vi "Test Set Active Funnel.vi"(8 "error in (no error)":errorcluster) -> (0 "error out":errorcluster)   [LabVIEW 2019]
uses:
  <vilib>/addons/_JKI Toolkits/Caraya/classes/Test/Test.lvclass
  <vilib>/addons/_JKI Toolkits/Caraya/classes/Assert/Assert.lvclass
  Setting Database/Setting Database.lvclass
  <vilib>/JKI/JKI SMO/SMO/SMO.lvclass
  C:/Program Files (x86)/National Instruments/LabVIEW 2019/vi.lib/JKI/JKI SMO/SMO/SMO.lvclass
  Funnel Settings/Funnel Settings.lvclass
  C:/Users/Albro/Documents/GitHub/AFM-Lithography/lvsrc/Classes/Settings/ObjectSettings/ObjectSettings.lvclass
  <vilib>/addons/_JKI Toolkits/Caraya/classes/Assert/Assert Equal Value_Variant.vi
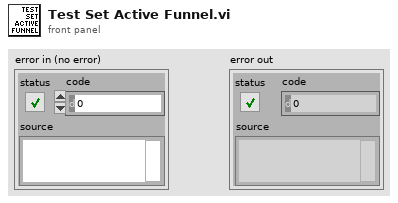
[diagram p1: front panel]
types:
  T1 = typedef "Setting Database.lvclass/PublicEvents--Cluster.ctl" = cluster{"NewActivePath":refnum<user-event>, "PathsUpdated":refnum<user-event>, "RectanglesUpdated":refnum<user-event>, "NewActiveRectangle":refnum<user-event>, "NewActiveFunnel":refnum<user-event>, "FunnelsUpdated":refnum<user-event>, "NewActiveDot":refnum<user-event>, "DotsUpdated":refnum<user-event>}
  T2 = typedef "Setting Database.lvclass/PrivateEvents--Setting Database.Refresh.ctl" = cluster{"Paths":string[], "Rectangles":string[], "Funnels":string[], "Dots":string[]}
  T3 = typedef "Setting Database.lvclass/PublicEvents--Setting Database.NewActiveFunnel.ctl" = refnum<class "Funnel Settings.lvclass">
  T4 = typedef "Setting Database.lvclass/PublicEvents--Setting Database.FunnelsUpdated.ctl" = refnum<class "Funnel Settings.lvclass">[]
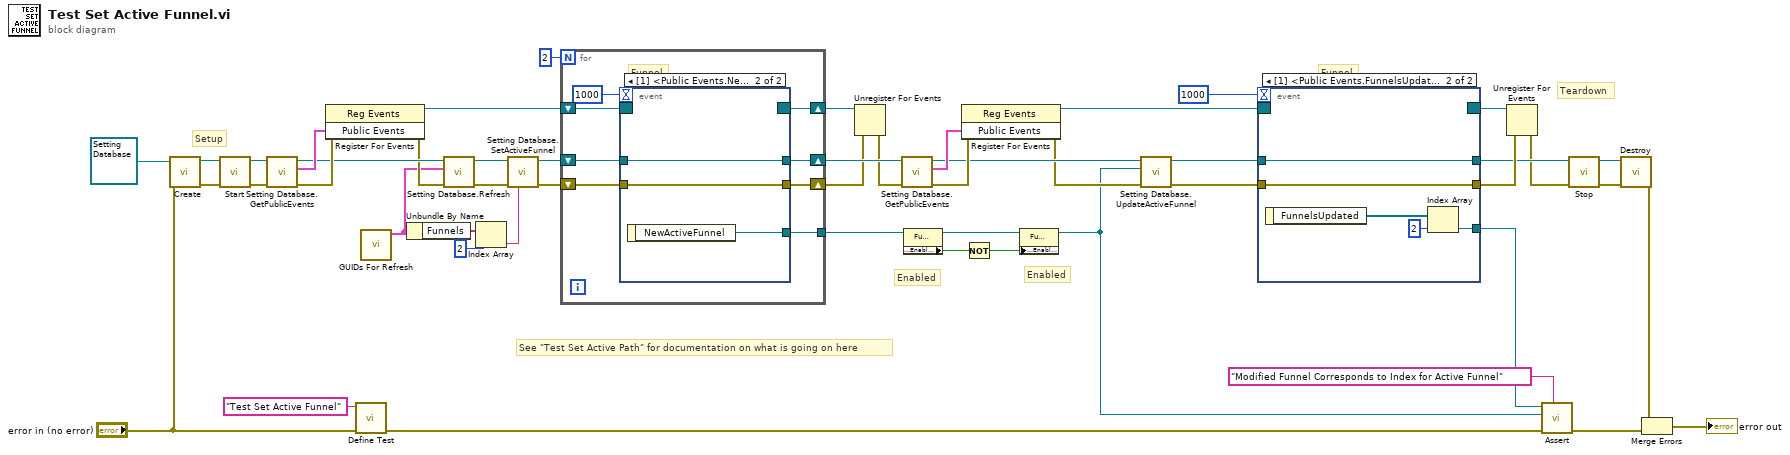
[diagram p0: block diagram]
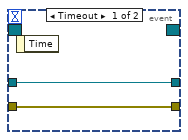
[diagram p2: hidden frame]
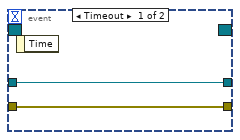
[diagram p3: hidden frame]
diagram:
  # "See \"Test Set Active Path\" for documentation on what is going on here"
  # "Enabled"
  # "Enabled"
  # "Funnel"
  # "Teardown"
  # "Setup"
  n1 = call <vilib>:"Create.vi"("error in (no error)"="error in (no error)", "SMO"=refnum<class "Setting Database.lvclass"> refnum ("Setting Database.lvclass")) -> ("error out"=w47:errorcluster, "SMO out"=w40:refnum<class "Setting Database.lvclass">)  [unwired: 7 in, 1 out]
  n2 = call <vilib>:"Start.vi"("error in (no error)"=w47, "SMO"=w40) -> ("error out"=w46:errorcluster, "SMO out"=w39:refnum<class "Setting Database.lvclass">)  [unwired: 8 in]
  n3 = call "Setting Database.GetPublicEvents.vi"("error in (no error)"=w46, "Setting Database"=w39) -> ("error out"=w44:errorcluster, "Public Events"=w36:T1, "Setting Database out"=w33:refnum<class "Setting Database.lvclass">)  [unwired: 7 in]
  n4 = register-events(error in=w44, w36) -> (reference out=w34:refnum<event-registration>, error out=w32:errorcluster)  [unwired: 1 in]
  n5 = call <vilib>:"Define Test.vi"("error in (no error)"="error in (no error)", "Label (VI Title)"="Test Set Active Funnel") -> ("error out"=w49:errorcluster)  [unwired: 8 in, 1 out]
  n6 = call "GUIDs For Refresh.vi"() -> ("Initialize"=w2:T2)  [unwired: 11 in]
  n7 = Unbundle By Name(w2) -> ("Funnels"=w4:string[])
  n8 = call "Setting Database.Refresh.vi"("error in (no error)"=w32, "Initialize"=w2, "Setting Database"=w33) -> ("error out"=w7:errorcluster, "Setting Database out"=w9:refnum<class "Setting Database.lvclass">)  [unwired: 7 in]
  n9 = Index Array(array=w4, index=2) -> (element=w1:string)
  n10 = call "Setting Database.SetActiveFunnel.vi"("error in (no error)"=w7, "SetActiveFunnel"=w1, "Setting Database"=w9) -> ("error out"=w6:errorcluster, "Setting Database out"=w8:refnum<class "Setting Database.lvclass">)  [unwired: 7 in]
  n11 = for {
    N: 2 -> [_]
    tunnel: [w53] -> w20
    shift-right: [w58] -> w37
    shift-left: w34 -> [w56]
    shift-right: [w55] -> w31
    shift-left: w8 -> [w52]
    shift-right: [w54] -> w30
    shift-left: w6 -> [w51]
    # "Funnel"
    n12 = event shown="[1] <Public Events.NewActiveFunnel>: User Event" {
      selector: w56 -> [_ _]
      dyn-events: [_ _] -> w58
      timeout: 1000 -> [_ _]
      tunnel: [w60 w63] -> w54
      tunnel: w51 -> [w60 w63]
      tunnel: w52 -> [w59 w62]
      tunnel: [w59 w62] -> w55
      tunnel: [_ w61] -> w53
      event Timeout {
        n13 = event-data() -> ()  [unwired: 1 in, 1 out]
      }
      event User Event {
        n14 = event-data() -> ("NewActiveFunnel"=w61:T3)  [unwired: 1 in]
      }
    }
  }
  n15 = Unregister For Events(event registration refnum=w37, error in=w30) -> (error out=w29:errorcluster)
  n16 = call "Setting Database.GetPublicEvents.vi"("error in (no error)"=w29, "Setting Database"=w31) -> ("error out"=w27:errorcluster, "Public Events"=w28:T1, "Setting Database out"=w14:refnum<class "Setting Database.lvclass">)  [unwired: 7 in]
  n17 = property on="Property Node" class="Funnel Settings.lvclass"(reference=w20) -> (reference out=w19:T3, "Accessors:Enabled"=w18:bool)  [unwired: 1 in, 1 out]
  n18 = register-events(error in=w27, w28) -> (reference out=w23:refnum<event-registration>, error out=w13:errorcluster)  [unwired: 1 in]
  n19 = Not(x=w18) -> (.not. x?=w17:bool)
  n20 = property on="Property Node" class="Funnel Settings.lvclass"(reference=w19, "Accessors:Enabled"=w17) -> (reference out=w10:T3)  [unwired: 1 in, 1 out]
  n21 = call "Setting Database.UpdateActiveFunnel.vi"("error in (no error)"=w13, "UpdateActiveFunnel"=w10, "Setting Database"=w14) -> ("error out"=w11:errorcluster, "Setting Database"=w12:refnum<class "Setting Database.lvclass">)  [unwired: 7 in]
  n22 = event shown="[1] <Public Events.FunnelsUpdated>: User Event" {
    selector: w23 -> [_ _]
    dyn-events: [_ _] -> w24
    timeout: 1000 -> [_ _]
    tunnel: [w65 w70] -> w26
    tunnel: w11 -> [w65 w70]
    tunnel: w12 -> [w64 w69]
    tunnel: [w64 w69] -> w22
    tunnel: [_ w67] -> w16
    event Timeout {
      n23 = event-data() -> ()  [unwired: 1 in, 1 out]
    }
    event User Event {
      n24 = event-data() -> ("FunnelsUpdated"=w68:T4)  [unwired: 1 in]
      n25 = Index Array(array=w68, index=2) -> (element=w67:refnum<class "Funnel Settings.lvclass">)
    }
  }
  n26 = Unregister For Events(event registration refnum=w24, error in=w26) -> (error out=w21:errorcluster)
  n27 = call-poly <vilib>:"Assert.vi"("Label"="Modified Funnel Corresponds to Index for Active Funnel", "error in (no error)"=w49, "Actual"=w10, "Expected"=w16) -> ("error out"=w50:errorcluster)  [unwired: 6 in, 1 out]
  n28 = call <vilib>:"Stop.vi"("error in (no error)"=w21, "SMO"=w22) -> ("error out"=w45:errorcluster, "SMO out"=w38:refnum<class "Setting Database.lvclass">)  [unwired: 8 in]
  n29 = call <vilib>:"Destroy.vi"("error in (no error)"=w45, "SMO"=w38) -> ("error out"=w43:errorcluster)  [unwired: 9 in]
  n30 = Merge Errors(w43, w50) -> (→"error out":errorcluster)
